vi "Main.vi"(10 "Name":string, 11 "Module Admin":refnum<class "Delacor_lib_QMH_Module Admin.lvclass">) -> ()   [LabVIEW 2023, in "Settings Master.lvlib"]
doc: "This template is based off of the Queued Message Handler design pattern and the Queued Message Handler project template that ships with LabVIEW.\n\nThe main difference is that the queue is private to this module and communication between modules is performed via Broadcast and Request events.\n\nRequest events are wrapped in public API methods and are handled in the Event Handling Loop (EHL) of this VI. Any module can register for Broadcast events sent by this module. The EHL generates messages based on user interface actions.\n\nThe Message Handling Loop (MHL) processes messages generated by the EHL, or by other messages. The messages are string values, so new messages can be added easily to the Message Cases case structure in the MHL. Each message cluster can also provide an optional value for Message Data, which is a variant that can be converted to whatever message-specific data is required.\n_____\nBased on DQMH Project Template 6.1.0.94."
uses:
  Settings Master.lvlib
  <vilib>/Delacor/Delacor QMH/Libraries/Message Queue_class/Delacor_lib_QMH_Message Queue.lvclass
  Module Data--cluster.ctl
  <vilib>/Utility/miscctls.llb/LVPointTypeDef.ctl
  <vilib>/Utility/error.llb/Error Cluster From Error Code.vi
  <vilib>/ErrorRing/Error Ring.xnode
  <vilib>/Delacor/Delacor QMH/Libraries/Message Queue_class/Delacor_lib_QMH_Enqueue Message (Single).vi
  Stop Argument--cluster.ctl
  <vilib>/Delacor/Delacor QMH/Libraries/Module Admin_class/Delacor_lib_QMH_Module Admin.lvclass
  <vilib>/Utility/config.llb/NI_LVConfig.lvlib
  <vilib>/Utility/sysdir.llb/System Directory Type.ctl
  Heat UI/Settings Type.ctl
  Get Settings (Reply Payload)--cluster.ctl
  Get Settings Argument--cluster.ctl
  Drive/Calc_Type.ctl
  Drive/Drive.lvlib
  Menu/Setts.ctl
  SubPanel Argument--cluster.ctl
panel:
  in  "Download Square":bool
  in  "Save Square":bool
  in  "Save":bool
  in  "Main":T4={"Heat"={"KPтерм"=8.0, "TNтерм"=12.0, "KPниз"=4.0, "TNниз"=8.0, "COM ADC"="", "COM Termex"="", "KPдд"=4.0, "TNдд"=8.0, "Multiper"=1.0}, "Расчёты"={"Vm0"=8.0, "aa"=8.0, "bb"=8.0, "K0"=8.0, "A"=8.0, "B"=8.0}, "Видеосистема"=FALSE, "Anton Paar"={"IP adress"="192.168.0.110"}, "MIDA COM"="COM11"} caption="Настройки" {"Расчёты"."B" min=0.0 max=150.0 format="%.8f"; "Расчёты"."A" min=0.0 max=150.0 format="%.8f"; "Расчёты"."K0" min=0.0 max=150.0 format="%.2f"; "Расчёты"."bb" min=0.0 max=150.0 format="%.8f"; "Расчёты"."aa" min=0.0 max=150.0 format="%.8f"; "Расчёты"."Vm0" min=0.0 max=150.0 format="%.2f"; "Heat"."Multiper" min=0.0 max=150.0 format="%.2f"; "Heat"."TNдд" min=0.0 max=150.0 format="%.2f"; "Heat"."KPдд" min=0.0 max=150.0 format="%.2f"; "Heat"."TNниз" min=0.0 max=150.0 format="%.2f"; "Heat"."KPниз" min=0.0 max=150.0 format="%.2f"; "Heat"."TNтерм" min=0.0 max=150.0 format="%.2f"; "Heat"."KPтерм" min=0.0 max=150.0 format="%.2f"}
  out "error out":errorcluster
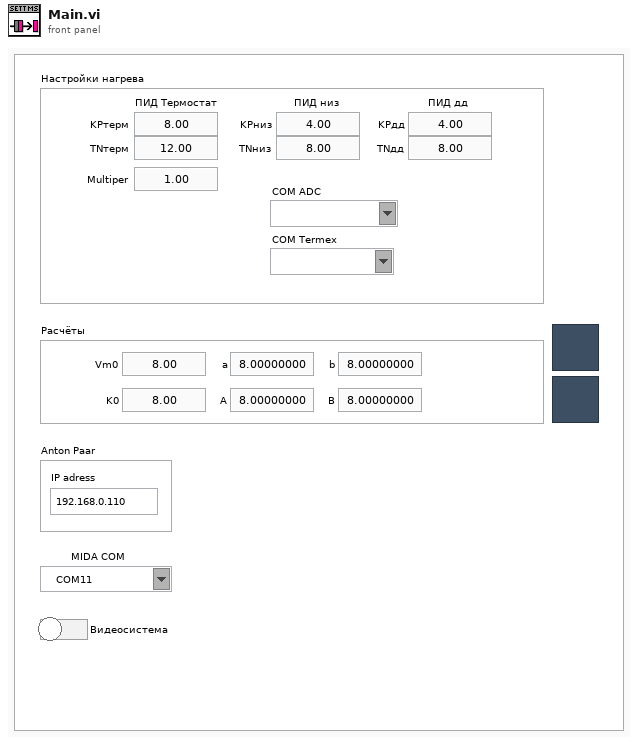
[diagram p1: front panel]
types:
  T1 = typedef "Heat UI.lvlib/Settings Type.ctl" = cluster{"KPтерм":dbl, "TNтерм":dbl, "KPниз":dbl, "TNниз":dbl, "COM ADC":refnum<visa-resource-name>, "COM Termex":refnum<visa-resource-name>, "KPдд":dbl, "TNдд":dbl, "Multiper":dbl}
  T2 = typedef "Drive.lvlib/Calc_Type.ctl" = cluster{"Vm0":dbl, "aa":dbl, "bb":dbl, "K0":dbl, "A":dbl, "B":dbl}
  T3 = typedef "Menu.lvlib/Setts.ctl" = cluster{"IP adress":string}
  T4 = cluster{"Heat":T1, "Расчёты":T2, "Видеосистема":bool, "Anton Paar":T3, "MIDA COM":refnum<visa-resource-name>}
  T5 = typedef "Settings Master.lvlib/Request Events--cluster.ctl" = cluster{"Stop Module":refnum<user-event>, "Show Panel":refnum<user-event>, "Hide Panel":refnum<user-event>, "Get Module Execution Status":refnum<user-event>, "Show Diagram":refnum<user-event>, "Get Settings":refnum<user-event>, "SubPanel":refnum<user-event>}
  T6 = typedef "Settings Master.lvlib/Module Data--cluster.ctl" = cluster{"Status":string, "ini path":path, "Main":cluster{"Heat":T1, "Расчёты":T2, "Видеосистема":bool, "Anton Paar":T3, "MIDA COM":refnum<visa-resource-name>}}
  T7 = enum32{"invalid lock state", "Not Locked", "Locked (No Password)", "Password-protected"}
  T8 = typedef "Settings Master.lvlib/Stop Argument--cluster.ctl" = cluster{"Origin":string, "Exit via Stop Module Req?":bool, "Wait for Module to stop?":bool}
  T9 = typedef "Settings Master.lvlib/Get Settings Argument--cluster.ctl" = cluster{"Wait Notifier":refnum<notifier>, "wait for reply":bool}
  T10 = typedef "Settings Master.lvlib/SubPanel Argument--cluster.ctl" = cluster{"Sub Panel":refnum<vi>}
  T11 = typedef "LVPointTypeDef.ctl" = cluster{"Horizontal":i16, "Vertical":i16}
  T12 = enum32{"Invalid", "Standard", "Closed", "Hidden", "Minimized", "Maximized"}
  T13 = typedef "Settings Master.lvlib/Get Settings (Reply Payload)--cluster.ctl" = cluster{"Main":cluster{"Heat":T1, "Расчёты":T2, "Видеосистема":bool, "Anton Paar":T3, "MIDA COM":refnum<visa-resource-name>}, "error":errorcluster}
  T14 = typedef "System Directory Type.ctl" = i32
  T15 = typedef "NI_LVConfig.lvlib/Config Data RefNum.ctl" = refnum<k1>
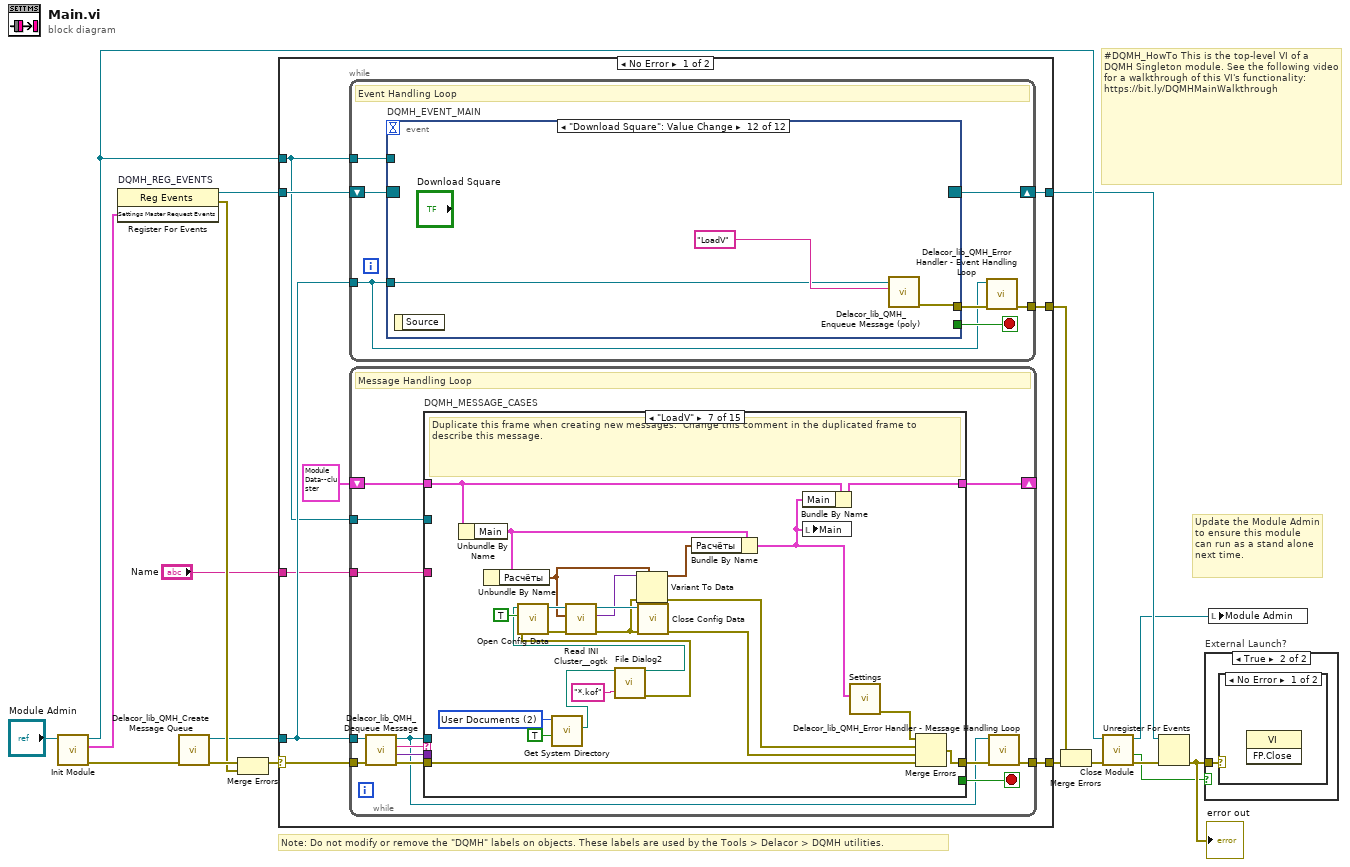
[diagram p0: block diagram]
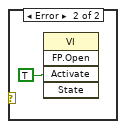
[diagram p3: hidden frame]
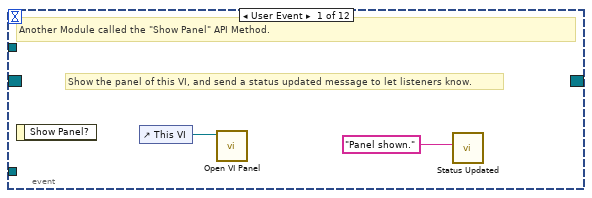
[diagram p4: hidden frame]
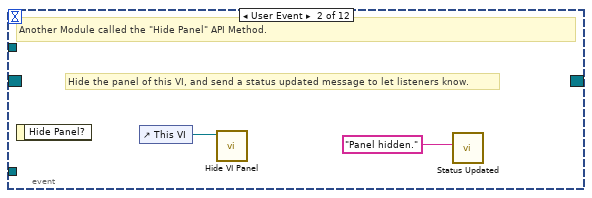
[diagram p5: hidden frame]
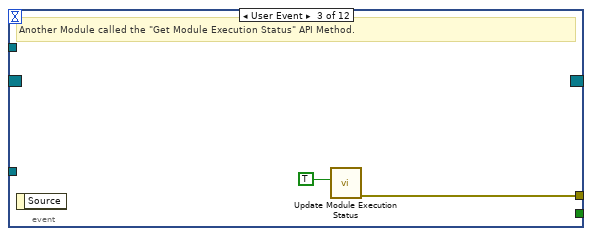
[diagram p6: hidden frame]
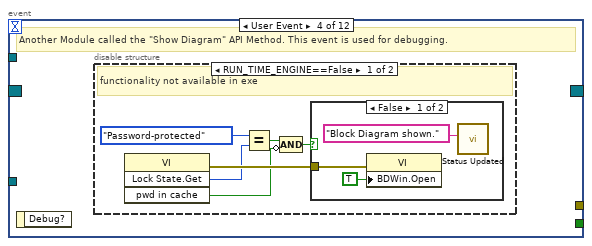
[diagram p7: hidden frame]
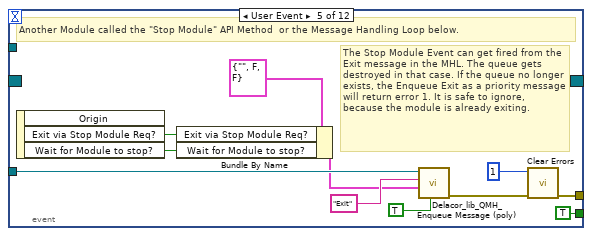
[diagram p10: hidden frame]
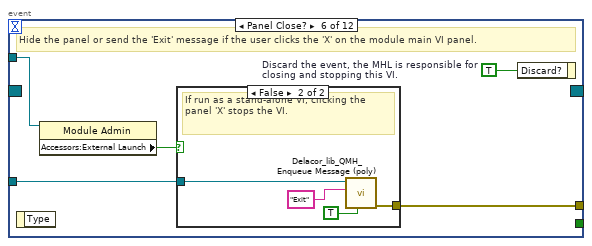
[diagram p11: hidden frame]
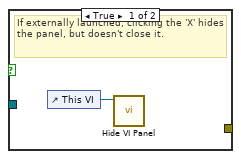
[diagram p12: hidden frame]
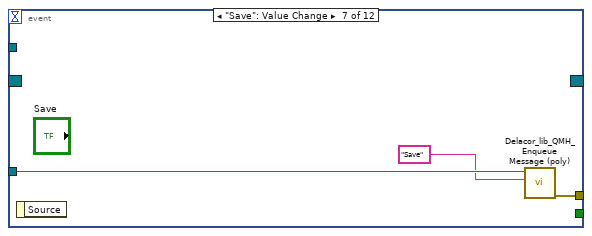
[diagram p13: hidden frame]
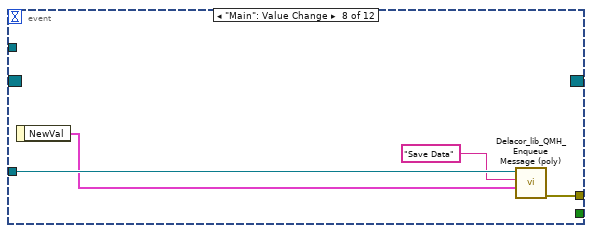
[diagram p14: hidden frame]
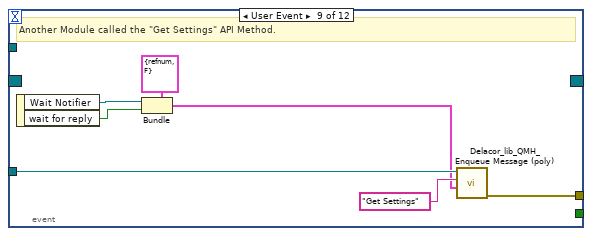
[diagram p15: hidden frame]
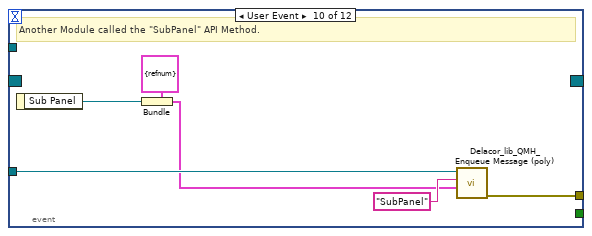
[diagram p16: hidden frame]
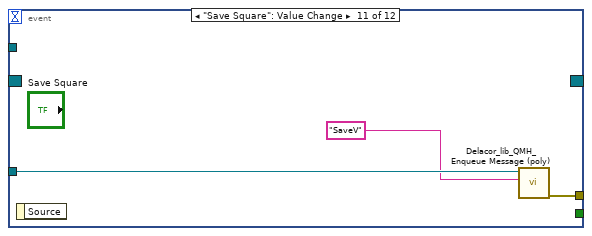
[diagram p17: hidden frame]
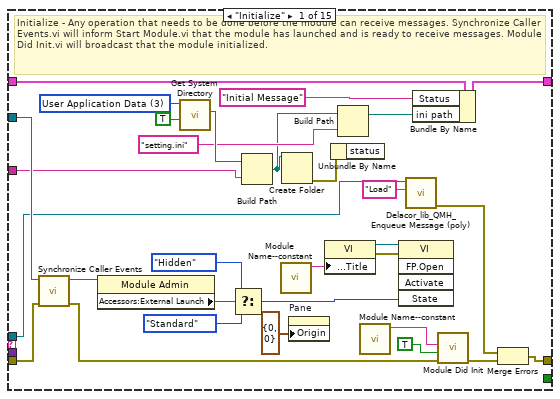
[diagram p18: hidden frame]
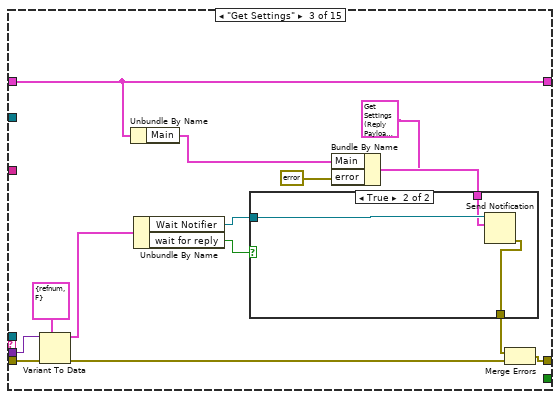
[diagram p20: hidden frame]
diagram:
  # "#DQMH_HowTo This is the top-level VI of a DQMH Singleton module. See the following video for a walkthrough of this VI's functionality: https://bit.ly/DQMHMainWalkthrough"
  # "Note: Do not modify or remove the \"DQMH\" labels on objects. These labels are used by the Tools > Delacor > DQMH utilities."
  # "Update the Module Admin to ensure this module can run as a stand alone next time."
  n1 = call "Init Module.vi"("Singleton Module Admin in"="Module Admin") -> ("error out"=w17:errorcluster, "Settings Master Request Events"=w6:T5, "Singleton Module Admin out"=w9:refnum<class "Delacor_lib_QMH_Module Admin.lvclass">)  [unwired: 8 in]
  n2 = register-events "DQMH_REG_EVENTS"(w6) -> (reference out=w7:refnum<event-registration>, error out=w10:errorcluster)  [unwired: 2 in]
  n3 = call <vilib>:"Delacor_lib_QMH_Create Message Queue.vi"("error in"=w17) -> ("error out"=w12:errorcluster, "Message Queue"=w5:refnum<class "Delacor_lib_QMH_Message Queue.lvclass">)  [unwired: 9 in]
  n4 = Merge Errors(w12, w10) -> (w11:errorcluster)
  n5 = case shown="No Error" w11 {
    selector: w11 -> [w25 w323]
    tunnel: [w27 w322] -> w18
    tunnel: [w24 w328] -> w8
    tunnel: w7 -> [w22 w328]
    tunnel: w5 -> [w21 w321]
    tunnel: [w26 _] -> w15
    tunnel: w9 -> [w20 w324]
    tunnel: "Name" -> [w19 _]
    frame No Error {
      n6 = while {
        tunnel: w21 -> [w28]
        shift-right: [w31] -> w24
        shift-left: w22 -> [w32]
        tunnel: [w33] -> w26
        tunnel: w20 -> [w29]
        stop <- w30 stop-if-true
        # "Event Handling Loop"
        n7 = event "DQMH_EVENT_MAIN" shown="[11] \"Download Square\": Value Change" {
          selector: w32 -> [_ _ _ _ _ _ _ _ _ _ _ _]
          dyn-events: [_ _ _ _ _ _ _ _ _ _ _ _] -> w31
          timeout: _ -> [_ _ _ _ _ _ _ _ _ _ _ _]
          tunnel: [_ _ _ _ TRUE ("Discard?") _ _ _ _ _ _ _] -> w30
          tunnel: w28 -> [_ _ _ _ w56 w63 w72 w76 w84 w90 w92 w94]
          tunnel: [_ _ w40 _ w59 w65 w73 w77 w78 w85 w93 w95] -> w34
          tunnel: w29 -> [_ _ _ _ _ w62 _ _ _ _ _ _]
          event User Event {
            # "Show the panel of this VI, and send a status updated message to let listeners know."
            # "Another Module called the \"Show Panel\" API Method."
            n8 = event-data() -> ()  [unwired: 1 in, 1 out]
            n9 = control-ref of="This VI"() -> (w36:refnum<vi>)
            n10 = call "Open VI Panel.vi"("VI"=w36) -> ()  [unwired: 10 in, 1 out]
            n11 = call "Status Updated.vi"("Status"="Panel shown." ("format string")) -> ()  [unwired: 10 in, 1 out]
          }
          event User Event {
            # "Hide the panel of this VI, and send a status updated message to let listeners know."
            # "Another Module called the \"Hide Panel\" API Method."
            n12 = event-data() -> ()  [unwired: 1 in, 1 out]
            n13 = control-ref of="This VI"() -> (w38:refnum<vi>)
            n14 = call "Hide VI Panel.vi"("VI"=w38) -> ()  [unwired: 10 in, 1 out]
            n15 = call "Status Updated.vi"("Status"="Panel hidden." ("format string")) -> ()  [unwired: 10 in, 1 out]
          }
          event User Event {
            # "Another Module called the \"Get Module Execution Status\" API Method."
            n16 = event-data() -> ()  [unwired: 1 in, 1 out]
            n17 = call "Update Module Execution Status.vi"("Running?"=TRUE) -> ("error out"=w40:errorcluster)  [unwired: 10 in]
          }
          event User Event {
            # "Another Module called the \"Show Diagram\" API Method. This event is used for debugging."
            n18 = event-data() -> ()  [unwired: 1 in, 1 out]
            n19 = disable-structure shown="RUN_TIME_ENGINE==False" {
              frame condition #0 (active) {
                # "functionality not available in exe"
                n20 = invoke class="VI" method="Lock State.Get"() -> (error out=w46:errorcluster, "Get Lock State"=w45:T7, "pwd in cache"=w42:bool)  [unwired: 4 in, 1 out]
                n21 = Equal?(x=T7."Password-protected", y=w45) -> (x = y?=w43:bool)
                n22 = Compound Arithmetic op=AND(w43, invert w42) -> (w41:bool)
                n23 = case shown="False" w41 {
                  tunnel: w46 -> [w49 _]
                  frame False {
                    n24 = property class="VI"(error in=w49, "BDWin.Open"=TRUE ("Block Diagram Window:Open")) -> ()  [unwired: 1 in, 2 out]
                    n25 = call "Status Updated.vi"("Status"="Block Diagram shown." ("format string")) -> ()  [unwired: 10 in, 1 out]
                  }
                  frame True {
                    # "Password-protected VI, and the password is not in the cache. Do not show the diagram."
                  }
                }
              }
              frame condition #1 {
              }
            }
          }
          event User Event {
            # "The Stop Module Event can get fired from the Exit message in the MHL. The queue gets destroyed in that case. If the queue no longer exists, the Enqueue Exit as a priority message will return error 1. It is safe to ignore, because the module is already exiting."
            # "Another Module called the \"Stop Module\" API Method  or the Message Handling Loop below."
            n26 = event-data() -> ("Exit via Stop Module Req?"=w52:bool, "Wait for Module to stop?"=w51:bool)  [unwired: 1 in, 1 out]
            n27 = Bundle By Name(cluster=T8 {"Origin"="", "Exit via Stop Module Req?"=FALSE, "Wait for Module to stop?"=FALSE} ("Stop Argument"), "Exit via Stop Module Req?"=w52, "Wait for Module to stop?"=w51) -> (w50:T8)
            n28 = call-poly <vilib>:"Delacor_lib_QMH_Enqueue Message (poly).vi"("Priority Message? (F)"=TRUE, "Message Data"=w50, "Message"="Exit", "Message Queue in"=w56) -> ("error out"=w60:errorcluster)  [unwired: 6 in, 1 out]
            n29 = call <vilib>:"Clear Errors.vi"("error in (no error)"=w60, "specific error code to clear (0: all)"=1) -> ("error out"=w59:errorcluster)  [unwired: 4 in, 1 out]
          }
          event Panel Close? {
            w64 = TRUE  # Discard the event, the MHL is responsible for closing and stopping this VI.
            # "Hide the panel or send the 'Exit' message if the user clicks the 'X' on the module main VI panel."
            n30 = event-data() -> ()  [unwired: 1 in, 1 out]
            n31 = property class="Module Admin"(reference=w62) -> ("Accessors:External Launch"=w61:bool)  [unwired: 1 in, 2 out]
            n32 = case shown="False" w61 {
              tunnel: w63 -> [_ w69]
              tunnel: [_ w70] -> w65
              frame True {
                # "If externally launched, clicking the 'X' hides the panel, but doesn't close it."
                n33 = control-ref of="This VI"() -> (w66:refnum<vi>)
                n34 = call "Hide VI Panel.vi"("VI"=w66) -> ()  [unwired: 10 in, 1 out]
              }
              frame False {
                # "If run as a stand-alone VI, clicking the panel 'X' stops the VI."
                n35 = call-poly <vilib>:"Delacor_lib_QMH_Enqueue Message (poly).vi"("Priority Message? (F)"=TRUE, "Message"="Exit", "Message Queue in"=w69) -> ("error out"=w70:errorcluster)  [unwired: 7 in, 1 out]
              }
            }
            n36 = event-data("Discard?"=w64) -> ()  [unwired: 1 in, 1 out]
          }
          event "Save": Value Change {
            n37 = event-data() -> ()  [unwired: 1 in, 1 out]
            n38 = call-poly <vilib>:"Delacor_lib_QMH_Enqueue Message (poly).vi"("Message"="Save", "Message Queue in"=w72) -> ("error out"=w73:errorcluster)  [unwired: 8 in, 1 out]
          }
          event "Main": Value Change {
            n39 = event-data() -> ("NewVal"=w75:T4)  [unwired: 1 in]
            n40 = call-poly <vilib>:"Delacor_lib_QMH_Enqueue Message (poly).vi"("Message Data"=w75, "Message"="Save Data", "Message Queue in"=w76) -> ("error out"=w77:errorcluster)  [unwired: 7 in, 1 out]
          }
          event User Event {
            # "Another Module called the \"Get Settings\" API Method."
            n41 = event-data() -> ("Wait Notifier"=w80:refnum<notifier>, "wait for reply"=w79:bool)  [unwired: 1 in]
            n42 = Bundle(cluster=T9 {"Wait Notifier"=refnum, "wait for reply"=FALSE} ("Get Settings Argument"), "Wait Notifier"=w80, "wait for reply"=w79) -> (w81:T9)
            n43 = call-poly <vilib>:"Delacor_lib_QMH_Enqueue Message (poly).vi"("Message Data"=w81, "Message"="Get Settings", "Message Queue in"=w84) -> ("error out"=w78:errorcluster)  [unwired: 7 in, 1 out]
          }
          event User Event {
            # "Another Module called the \"SubPanel\" API Method."
            n44 = event-data() -> ("Sub Panel"=w86:refnum<vi>)  [unwired: 1 in]
            n45 = Bundle(cluster=T10 {"Sub Panel"=refnum} ("SubPanel Argument"), "Sub Panel"=w86) -> (w87:T10)
            n46 = call-poly <vilib>:"Delacor_lib_QMH_Enqueue Message (poly).vi"("Message Data"=w87, "Message"="SubPanel", "Message Queue in"=w90) -> ("error out"=w85:errorcluster)  [unwired: 7 in, 1 out]
          }
          event "Save Square": Value Change {
            n47 = event-data() -> ()  [unwired: 1 in, 1 out]
            n48 = call-poly <vilib>:"Delacor_lib_QMH_Enqueue Message (poly).vi"("Message"="SaveV", "Message Queue in"=w92) -> ("error out"=w93:errorcluster)  [unwired: 8 in, 1 out]
          }
          event "Download Square": Value Change {
            n49 = event-data() -> ()  [unwired: 1 in, 1 out]
            n50 = call-poly <vilib>:"Delacor_lib_QMH_Enqueue Message (poly).vi"("Message"="LoadV", "Message Queue in"=w94) -> ("error out"=w95:errorcluster)  [unwired: 8 in, 1 out]
          }
        }
        n51 = call-dynamic "Delacor_lib_QMH_Error Handler - Event Handling Loop.vi"("error in"=w34, "Message Queue in"=w28) -> ("dup error in"=w33:errorcluster)  [unwired: 8 in, 1 out]
      }
      n52 = while {
        tunnel: w21 -> [w100]
        shift-right: [w104] -> _
        shift-left: T6 {"Status"="", "ini path"=path "", "Main"={"Heat"={"KPтерм"=8.0, "TNтерм"=12.0, "KPниз"=4.0, "TNниз"=8.0, "COM ADC"="", "COM Termex"="", "KPдд"=4.0, "TNдд"=8.0, "Multiper"=1.0}, "Расчёты"={"Vm0"=8.0, "aa"=8.0, "bb"=8.0, "K0"=8.0, "A"=8.0, "B"=8.0}, "Видеосистема"=FALSE, "Anton Paar"={"IP adress"="192.168.0.110"}, "MIDA COM"="COM11"}} ("Data Cluster") -> [w105]
        tunnel: w25 -> [w108]
        tunnel: [w106] -> w27
        tunnel: w20 -> [w98]
        tunnel: w19 -> [w97]
        stop <- w103 stop-if-true
        # "Message Handling Loop"
        n53 = call-dynamic "Delacor_lib_QMH_Dequeue Message.vi"("error in"=w108, "Message Queue in"=w100) -> ("error out"=w107:errorcluster, "Message Data"=w101:variant, "Message"=w102:string, "Message Queue out"=w99:refnum<class "Delacor_lib_QMH_Message Queue.lvclass">)  [unwired: 6 in]
        n54 = case "DQMH_MESSAGE_CASES" shown="\"LoadV\"" w102 {
          selector: w102 -> [_ _ _ _ _ _ _ _ _ _ _ _ _ _ w308]
          tunnel: w99 -> [w117 _ _ _ _ _ _ _ _ _ _ _ w270 w300 _]
          tunnel: w107 -> [w138 w141 w155 w168 w171 w187 w210 w221 w237 w244 w255 w260 w277 w306 w310]
          tunnel: [w119 w141 w146 w160 w170 w186 w209 w220 w236 w253 w255 w259 w273 w303 w311] -> w109
          tunnel: w105 -> [w128 w140 w144 w167 w169 w185 w208 w214 w230 w247 w254 w257 w272 w285 w309]
          tunnel: [w127 w140 w144 w167 w169 w176 w201 w214 w230 w241 w254 w257 w272 w285 w309] -> w104
          tunnel: [_ _ _ _ _ _ _ _ _ _ _ _ _ w299 _] -> w103
          tunnel: w101 -> [_ _ w153 w165 _ _ _ _ _ w243 _ _ w271 w298 _]
          tunnel: w98 -> [w129 _ _ _ _ _ _ _ _ _ _ _ w269 w293 _]
          tunnel: w97 -> [w113 _ _ _ _ _ _ _ _ _ _ _ _ _ _]
          frame "Initialize" {
            w121 = T14 3 items=["User Home"=0, "User Desktop"=1, "User Documents"=2, "User Application Data"=3, "User Preferences"=4, "User Temporary"=5, "Public Documents"=6, "Public Application Data"=7, "Public Preferences"=8, "Public Cache"=13, "System Core Libraries"=9, "System Installed Libraries"=10, "Application Files"=11, "Boot Volume Root"=12] ("system directory type")
            # "Initialize - Any operation that needs to be done before the module can receive messages. Synchronize Caller Events.vi will inform Start Module.vi that the module has launched and is ready to receive messages. Module Did Init.vi will broadcast that the module initialized."
            n55 = call "Synchronize Caller Events.vi"("error in (no error)"=w138, "Singleton Module Admin in"=w129) -> ("error out"=w137:errorcluster, "Singleton Module Admin out"=w124:refnum<class "Delacor_lib_QMH_Module Admin.lvclass">)  [unwired: 8 in]
            n56 = property class="Module Admin"(reference=w124) -> ("Accessors:External Launch"=w133:bool)  [unwired: 1 in, 2 out]
            n57 = call <vilib>:"Get System Directory.vi"("create directory if not found? (F)"=TRUE, "system directory type"=w121) -> ("system directory"=w114:path)  [unwired: 9 in]
            n58 = Select(t=T12."Hidden" ("State"), s=w133, f=T12."Standard" ("State")) -> (s? t:f=w130:T12)
            n59 = Build Path(base path=w114, name or relative path=w113) -> (appended path=w110:path)
            n60 = call "Module Name--constant.vi"() -> ("Module Name"=w135:string)  [unwired: 11 in]
            n61 = Create Folder(path (use dialog)=w110) -> (error out=w112:errorcluster)  [unwired: 2 in, 2 out]
            n62 = property on="Pane" class="Pane"("Origin"=T11 {"Horizontal"=0, "Vertical"=0}) -> ()  [unwired: 2 in, 2 out]
            n63 = property class="VI"("Front Panel.Title"=w135) -> (reference out=w134:refnum<vi>, error out=w139:errorcluster)  [unwired: 2 in]
            n64 = Unbundle By Name(w112) -> ()  [unwired: 1 out]
            n65 = Build Path(base path=w110, name or relative path="setting.ini" ("string")) -> (appended path=w115:path)
            n66 = call "Module Name--constant.vi"() -> ("Module Name"=w125:string)  [unwired: 11 in]
            n67 = invoke class="VI" method="FP.Open"(reference=w134, error in=w139, "State"=w130) -> ()  [unwired: 2 in, 5 out]
            n68 = call-poly <vilib>:"Delacor_lib_QMH_Enqueue Message (poly).vi"("Message"="Load", "Message Queue in"=w117) -> ("error out"=w118:errorcluster)  [unwired: 8 in, 1 out]
            n69 = Bundle By Name(cluster=w128, "Status"="Initial Message" ("Initial Message"), "ini path"=w115) -> (w127:T6)
            n70 = call "Module Did Init.vi"("error in (no error)"=w137, "Initialized?"=TRUE, "Origin"=w125) -> ("error out"=w136:errorcluster)  [unwired: 8 in]
            n71 = Merge Errors(w118, w136) -> (w119:errorcluster)
          }
          frame "---Module Specific---" {
            # "Separator -- The following cases handle messages specific to this Module."
          }
          frame "Get Settings" {
            n72 = Variant To Data(error in=w155, type=T9 {"Wait Notifier"=refnum, "wait for reply"=FALSE} ("Get Settings Argument"), Variant=w153) -> (data=w151:T9, error out=w154:errorcluster)
            n73 = Unbundle By Name(w144) -> ("Main"=w143:T4)
            n74 = Unbundle By Name(w151) -> ("Wait Notifier"=w150:refnum<notifier>, "wait for reply"=w149:bool)
            n75 = Bundle By Name(cluster=T13 {"Main"={"Heat"={"KPтерм"=8.0, "TNтерм"=12.0, "KPниз"=4.0, "TNниз"=8.0, "COM ADC"="", "COM Termex"="", "KPдд"=4.0, "TNдд"=8.0, "Multiper"=1.0}, "Расчёты"={"Vm0"=8.0, "aa"=8.0, "bb"=8.0, "K0"=8.0, "A"=8.0, "B"=8.0}, "Видеосистема"=FALSE, "Anton Paar"={"IP adress"="192.168.0.110"}, "MIDA COM"="COM11"}, "error"={"status"=FALSE, "code"=0, "source"=""}} ("Get Settings (Reply Payload)"), "Main"=w143, "error"=errorcluster {"status"=FALSE, "code"=0, "source"=""}) -> (w148:T13)
            n76 = case shown="True" w149 {
              tunnel: w150 -> [_ w158]
              tunnel: w148 -> [_ w157]
              tunnel: [_ w156] -> w142
              frame False {
              }
              frame True {
                n77 = Send Notification(notification=w157, notifier=w158) -> (error out=w156:errorcluster)  [unwired: 1 in, 1 out]
              }
            }
            n78 = Merge Errors(w142, w154) -> (w146:errorcluster)
          }
          frame "SubPanel" {
            n79 = Variant To Data(error in=w168, type=T10 {"Sub Panel"=refnum} ("SubPanel Argument"), Variant=w165) -> (data=w163:T10, error out=w166:errorcluster)
            n80 = Unbundle By Name(w163) -> ("Sub Panel"=w161:refnum<vi>)
            n81 = control-ref of="This VI"() -> (w162:refnum<vi>)
            n82 = call "Insert SubPanel.vi"("VI Ref"=w162, "Subpanel Ref"=w161) -> ("error out"=w159:errorcluster)  [unwired: 9 in]
            n83 = Merge Errors(w159, w166) -> (w160:errorcluster)
          }
          frame "---Copy This Frame---" {
            # "Duplicate this frame when creating new messages.  Change this comment in the duplicated frame to describe this message."
            n84 = Merge Errors(w171) -> (w170:errorcluster)
          }
          frame "Load" {
            # "Duplicate this frame when creating new messages.  Change this comment in the duplicated frame to describe this message."
            n85 = Unbundle By Name(w185) -> ("Main"=w177:T4, "ini path"=w184:path)
            n86 = call <vilib>:"Open Config Data.vi"("create file if necessary (T)"=TRUE, "configuration file path"=w184) -> ("error out"=w182:errorcluster, "refnum"=w183:T15)  [unwired: 7 in, 1 out]
            n87 = call <userlib>:"Read INI Cluster__ogtk.vi"("error in (no error)"=w182, "INI Fomatted Cluster Type"=w177, "refnum"=w183) -> ("error out"=w179:errorcluster, "INI Fomatted Cluster"=w178:variant, "dup refnum"=w181:T15)  [unwired: 4 in, 2 out]
            n88 = call <vilib>:"Close Config Data.vi"("error in (no error)"=w179, "refnum"=w181) -> ("error out"=w180:errorcluster)  [unwired: 8 in, 1 out]
            n89 = Variant To Data(error in=w179, type=w177, Variant=w178) -> (data=w172:T4, error out=w175:errorcluster)
            n90 = Bundle By Name(cluster=w185, "Main"=w172) -> (w176:T6)
            n91 = local write "Main"(w172) -> ()
            n92 = call "Settings.vi"("Main"=w172) -> ("error out"=w173:errorcluster)  [unwired: 10 in]
            n93 = Merge Errors(w173, w175, w180, w187) -> (w186:errorcluster)
          }
          frame "LoadV" {
            w190 = T14 2 items=["User Home"=0, "User Desktop"=1, "User Documents"=2, "User Application Data"=3, "User Preferences"=4, "User Temporary"=5, "Public Documents"=6, "Public Application Data"=7, "Public Preferences"=8, "Public Cache"=13, "System Core Libraries"=9, "System Installed Libraries"=10, "Application Files"=11, "Boot Volume Root"=12] ("system directory type")
            # "Duplicate this frame when creating new messages.  Change this comment in the duplicated frame to describe this message."
            n94 = Unbundle By Name(w208) -> ("Main"=w196:T4)
            n95 = Unbundle By Name(w196) -> ("Расчёты"=w197:T2)
            n96 = call <vilib>:"Get System Directory.vi"("create directory if not found? (F)"=TRUE, "system directory type"=w190) -> ("system directory"=w188:path)  [unwired: 9 in]
            n97 = call "File Dialog2"("start path"=w188, "pattern (all files)"="*.kof") -> ("selected path"=w192:path, "error out"=w191:errorcluster)  [unwired: 10 in, 2 out]
            n98 = call <vilib>:"Open Config Data.vi"("error in (no error)"=w191, "create file if necessary (T)"=TRUE, "configuration file path"=w192) -> ("error out"=w206:errorcluster, "refnum"=w207:T15)  [unwired: 6 in, 1 out]
            n99 = call <userlib>:"Read INI Cluster__ogtk.vi"("error in (no error)"=w206, "INI Fomatted Cluster Type"=w197, "refnum"=w207) -> ("error out"=w203:errorcluster, "INI Fomatted Cluster"=w202:variant, "dup refnum"=w205:T15)  [unwired: 4 in, 2 out]
            n100 = Variant To Data(error in=w203, type=w197, Variant=w202) -> (data=w195:T2, error out=w200:errorcluster)
            n101 = call <vilib>:"Close Config Data.vi"("error in (no error)"=w203, "refnum"=w205) -> ("error out"=w204:errorcluster)  [unwired: 8 in, 1 out]
            n102 = Bundle By Name(cluster=w196, "Расчёты"=w195) -> (w194:T4)
            n103 = Bundle By Name(cluster=w208, "Main"=w194) -> (w201:T6)
            n104 = local write "Main"(w194) -> ()
            n105 = call "Settings.vi"("Main"=w194) -> ("error out"=w198:errorcluster)  [unwired: 10 in]
            n106 = Merge Errors(w198, w200, w204, w210) -> (w209:errorcluster)
          }
          frame "Save" {
            # "Duplicate this frame when creating new messages.  Change this comment in the duplicated frame to describe this message."
            n107 = Unbundle By Name(w214) -> ("ini path"=w213:path, "Main"=w211:T4)
            n108 = call <vilib>:"Open Config Data.vi"("create file if necessary (T)"=TRUE, "configuration file path"=w213) -> ("error out"=w218:errorcluster, "refnum"=w219:T15)  [unwired: 7 in, 1 out]
            n109 = call <userlib>:"Write INI Cluster__ogtk.vi"("error in (no error)"=w218, "INI Fomatted Cluster"=w211, "refnum"=w219) -> ("error out"=w216:errorcluster, "dup refnum"=w217:T15)  [unwired: 7 in]
            n110 = call <vilib>:"Close Config Data.vi"("error in (no error)"=w216, "refnum"=w217) -> ("error out"=w215:errorcluster)  [unwired: 8 in, 1 out]
            n111 = Merge Errors(w215, w221) -> (w220:errorcluster)
          }
          frame "SaveV" {
            w225 = T14 2 items=["User Home"=0, "User Desktop"=1, "User Documents"=2, "User Application Data"=3, "User Preferences"=4, "User Temporary"=5, "Public Documents"=6, "Public Application Data"=7, "Public Preferences"=8, "Public Cache"=13, "System Core Libraries"=9, "System Installed Libraries"=10, "Application Files"=11, "Boot Volume Root"=12] ("system directory type")
            # "Duplicate this frame when creating new messages.  Change this comment in the duplicated frame to describe this message."
            n112 = Unbundle By Name(w230) -> ("Main.Расчёты"=w228:T2)
            n113 = call <vilib>:"Get System Directory.vi"("create directory if not found? (F)"=TRUE, "system directory type"=w225) -> ("system directory"=w223:path)  [unwired: 9 in]
            n114 = call "File Dialog"("start path"=w223, "pattern (all files)"="*.kof") -> ("selected path"=w227:path, "error out"=w222:errorcluster)  [unwired: 10 in, 2 out]
            n115 = call <vilib>:"Open Config Data.vi"("error in (no error)"=w222, "create file if necessary (T)"=TRUE, "configuration file path"=w227) -> ("error out"=w234:errorcluster, "refnum"=w235:T15)  [unwired: 6 in, 1 out]
            n116 = call <userlib>:"Write INI Cluster__ogtk.vi"("error in (no error)"=w234, "INI Fomatted Cluster"=w228, "refnum"=w235) -> ("error out"=w232:errorcluster, "dup refnum"=w233:T15)  [unwired: 7 in]
            n117 = call <vilib>:"Close Config Data.vi"("error in (no error)"=w232, "refnum"=w233) -> ("error out"=w231:errorcluster)  [unwired: 8 in, 1 out]
            n118 = Merge Errors(w231, w237) -> (w236:errorcluster)
          }
          frame "Save Data" {
            # "Duplicate this frame when creating new messages.  Change this comment in the duplicated frame to describe this message."
            n119 = Variant To Data(error in=w244, type="Main", Variant=w243) -> (data=w239:T4, error out=w242:errorcluster)
            n120 = Unbundle By Name(w247) -> ("ini path"=w246:path)
            n121 = call <vilib>:"Open Config Data.vi"("create file if necessary (T)"=TRUE, "configuration file path"=w246) -> ("error out"=w251:errorcluster, "refnum"=w252:T15)  [unwired: 7 in, 1 out]
            n122 = call <userlib>:"Write INI Cluster__ogtk.vi"("error in (no error)"=w251, "INI Fomatted Cluster"=w239, "refnum"=w252) -> ("error out"=w249:errorcluster, "dup refnum"=w250:T15)  [unwired: 7 in]
            n123 = Bundle By Name(cluster=w247, "Main"=w239) -> (w241:T6)
            n124 = call <vilib>:"Close Config Data.vi"("error in (no error)"=w249, "refnum"=w250) -> ("error out"=w248:errorcluster)  [unwired: 8 in, 1 out]
            n125 = call "Settings.vi"("Main"=w239) -> ("error out"=w238:errorcluster)  [unwired: 10 in]
            n126 = Merge Errors(w238, w248, w242) -> (w253:errorcluster)
          }
          frame "---Exit and Error Handling---" {
            # "Separator - The following cases handle errors and exit messages."
          }
          frame "Simulate MHL Error" {
            # "#DQMH_HowTo The 'Simulate MHL Error' button  illustrates how the MHL handles errors. This event is instructional in nature and can be removed."
            # "Simulate an error occurring at the MHL"
            n127 = call "Module Name--constant.vi"() -> ("Module Name"=w256:string)  [unwired: 11 in]
            n128 = xnode "Error Ring"("parameter 0"=w256) -> ("error out"=w258:errorcluster)
            n129 = Merge Errors(w260, w258) -> (w259:errorcluster)
          }
          frame "Error" {
            # "#CodeRecommended - If you ever change the name of this \"Error\" message, you'll need to update the name in the Check Loop Error.vi as well."
            # "#CodeRecommended - If the module is running in standalone mode (External Launch = FALSE), this code will pop up an error dialog and call the 'Exit' message if an error occurs. Add more fine-grained error handling here."
            # "Error - Check the error message data and respond accordingly. This message is sent by the \"Error Handler\" VIs at the end of each loop in this application."
            n130 = property class="Module Admin"(reference=w269) -> ("Accessors:External Launch"=w268:bool)  [unwired: 1 in, 2 out]
            n131 = Variant To Data(error in=w277, type=errorcluster {"status"=FALSE, "code"=0, "source"=""} ("error constant"), Variant=w271) -> (data=w278:errorcluster, error out=w275:errorcluster)
            n132 = call "Error Reported.vi"("Error"=w278) -> ()  [unwired: 10 in, 1 out]
            n133 = case shown="False" w268 {
              tunnel: [w283 _] -> w274
              tunnel: w270 -> [w281 _]
              tunnel: w278 -> [w282 _]
              frame False {
                # "If the module is running standalone, then pop up an error dialog and call the \"Exit\" message."
                n134 = call <vilib>:"Simple Error Handler.vi"("error in (no error)"=w282) -> ()  [unwired: 4 in, 5 out]
                n135 = call-poly <vilib>:"Delacor_lib_QMH_Enqueue Message (poly).vi"("Priority Message? (F)"=TRUE, "Message"="Exit", "Message Queue in"=w281) -> ("error out"=w283:errorcluster)  [unwired: 7 in, 1 out]
              }
              frame True {
                # "If the module was launched externally, calling the Error Reported broadcast VI is the only action performed by the \"Error\" message. The module's caller can then process the error appropriately."
              }
            }
            n136 = Merge Errors(w275, w274) -> (w273:errorcluster)
            n137 = local write "error out"(w273) -> ()
          }
          frame "Exit" {
            w297 = 91  # 91: not all Exit messages will have an argument
            w299 = TRUE  # Stop the VI
            # "Release the message queue reference"
            # "Exit - Exit the application."
            n138 = Variant To Data(error in=w306, type=T8 {"Origin"="", "Exit via Stop Module Req?"=FALSE, "Wait for Module to stop?"=FALSE} ("Stop Argument"), Variant=w298) -> (data=w295:T8, error out=w302:errorcluster)
            n139 = Unbundle By Name(w285) -> ("ini path"=w288:path, "Main"=w286:T4)
            n140 = call <vilib>:"Clear Errors.vi"("error in (no error)"=w302, "specific error code to clear (0: all)"=w297) -> ("error out"=w305:errorcluster)  [unwired: 4 in, 1 out]
            n141 = call <vilib>:"Open Config Data.vi"("create file if necessary (T)"=TRUE, "configuration file path"=w288) -> ("error out"=w291:errorcluster, "refnum"=w292:T15)  [unwired: 7 in, 1 out]
            n142 = control-ref of="This VI"() -> (w294:refnum<vi>)
            n143 = call <userlib>:"Write INI Cluster__ogtk.vi"("error in (no error)"=w291, "INI Fomatted Cluster"=w286, "refnum"=w292) -> ("error out"=w289:errorcluster, "dup refnum"=w290:T15)  [unwired: 7 in]
            n144 = call <vilib>:"Close Config Data.vi"("error in (no error)"=w289, "refnum"=w290) -> ("error out"=w284:errorcluster)  [unwired: 8 in, 1 out]
            n145 = call-dynamic "Delacor_lib_QMH_Release Message Queue.vi"("error in"=w305, "Message Queue"=w300) -> ("error out"=w304:errorcluster)  [unwired: 9 in]
            n146 = call "Handle Exit.vi"("Stop Argument"=w295, "Admin in"=w293, "VI reference"=w294) -> ("error out"=w301:errorcluster)  [unwired: 7 in, 1 out]
            n147 = Merge Errors(w284, w304, w301) -> (w303:errorcluster)
          }
          frame Default {
            # "'Default' case only runs if there is a message that isn't defined in any of the other cases.  Output a programming error."
            n148 = call "Module Name--constant.vi"() -> ("Module Name"=w307:string)  [unwired: 11 in]
            n149 = xnode "Error Ring"("parameter 0"=w308, "parameter 1"=w307) -> ("error out"=w312:errorcluster)
            n150 = Merge Errors(w310, w312) -> (w311:errorcluster)
          }
        }
        n151 = call-dynamic "Delacor_lib_QMH_Error Handler - Message Handling Loop.vi"("error in"=w109, "Message Queue in"=w99) -> ("dup error in"=w106:errorcluster)  [unwired: 8 in, 1 out]
      }
    }
    frame Error {
      # "Synchronize Caller Events.vi will inform Start Module.vi that the module has launched and will let the code calling Start Module.vi register for broadcasts and would permit the caller receive the broadcast that an error occurred at launch time."
      n152 = call-dynamic "Delacor_lib_QMH_Release Message Queue.vi"("error in"=w323, "Message Queue"=w321) -> ("error out"=w322:errorcluster)  [unwired: 9 in]
      n153 = call "Synchronize Caller Events.vi"("Singleton Module Admin in"=w324) -> ("error out"=w329:errorcluster)  [unwired: 9 in, 1 out]
      n154 = call "Module Name--constant.vi"() -> ("Module Name"=w327:string)  [unwired: 11 in]
      n155 = Format Into String(format string="An error occurred during initialization. %s is no longer running.", w327) -> (resulting string=w325:string)  [unwired: 2 in, 1 out]
      n156 = Merge Errors(w322, w329) -> (w330:errorcluster)
      n157 = call "Error Reported.vi"("Additional Information"=w325, "Error"=w330) -> ()  [unwired: 9 in, 1 out]
    }
  }
  n158 = Merge Errors(w15, w18) -> (w14:errorcluster)
  n159 = call "Close Module.vi"("error in (no error)"=w14, "Module Admin in"=w9) -> ("error out"=w16:errorcluster, "External Launch"=w2:bool, "Module Admin out"=w3:refnum<class "Delacor_lib_QMH_Module Admin.lvclass">)  [unwired: 7 in]
  n160 = Unregister For Events(event registration refnum=w8, error in=w16) -> (error out=w13:errorcluster)
  "error out" <- w13
  n161 = case "External Launch?" shown="True" w2 {
    tunnel: w13 -> [_ w331]
    frame False {
    }
    frame True {
      n162 = case shown="No Error" w331 {
        frame No Error {
          n163 = invoke class="VI" method="FP.Close"() -> ()  [unwired: 3 in, 3 out]
        }
        frame Error {
          n164 = invoke class="VI" method="FP.Open"("Activate"=TRUE ("Activate?")) -> ()  [unwired: 4 in, 5 out]
        }
      }
    }
  }
  n165 = local write "Module Admin"(w3) -> ()
